vi "Rescale.vi"(4 "Max In":dbl=5.0, 5 "Max Out":dbl=1.0, 6 "Min In":dbl=5.0, 7 "Min Out":dbl=-1.0, 9 "Limit? (t)":bool=TRUE, 11 "Input":dbl=5.0 format="%#_13g") -> (3 "Output":dbl)   [LabVIEW 2013]
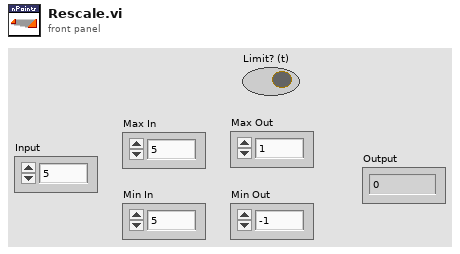
[diagram p1: front panel]
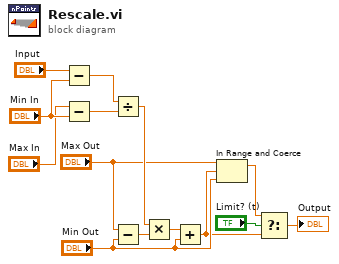
[diagram p0: block diagram]
diagram:
  n1 = Subtract(x="Input", y="Min In") -> (x-y=w10:dbl)
  n2 = Subtract(x="Max In", y="Min In") -> (x-y=w11:dbl)
  n3 = Divide(x=w10, y=w11) -> (x/y=w13:dbl)
  n4 = Subtract(x="Max Out", y="Min Out") -> (x-y=w12:dbl)
  n5 = Multiply(x=w13, y=w12) -> (x*y=w14:dbl)
  n6 = Add(x=w14, y="Min Out") -> (x+y=w4:dbl)
  n7 = In Range and Coerce(upper limit="Max Out", x=w4, lower limit="Min Out") -> (coerced(x)=w3:dbl)  [unwired: 1 out]
  n8 = Select(t=w3, s="Limit? (t)", f=w4) -> (s? t:f=→"Output":dbl)
